vi "SetActiveScanFunc.vi"(4 "FuncIndex":i32, 6 "SingleParMode":bool, 8 "error in (no error)":errorcluster caption="entrée d'erreur (pas d'erreur)", 9 "ScanTag":string, 10 "ScanTreeRef":refnum<vi>, 11 "Experiment en entrée":refnum<class "Experiment.lvclass"> caption="DNL_LabVIEW Object in") -> (0 "error out":errorcluster caption="sortie d'erreur", 1 "DesactivatedSPM":bool, 2 "SingleParModeOut":bool, 3 "Experiment en sortie":refnum<class "Experiment.lvclass"> caption="DNL_LabVIEW Object out")   [LabVIEW 2019, in "Experiment.lvclass"]
uses:
  Experiment.lvclass
  Experiment.lvclass/Experiment.ctl
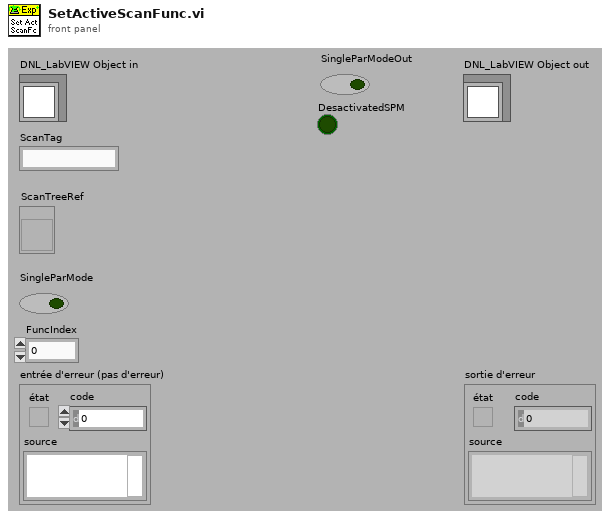
[diagram p1: front panel]
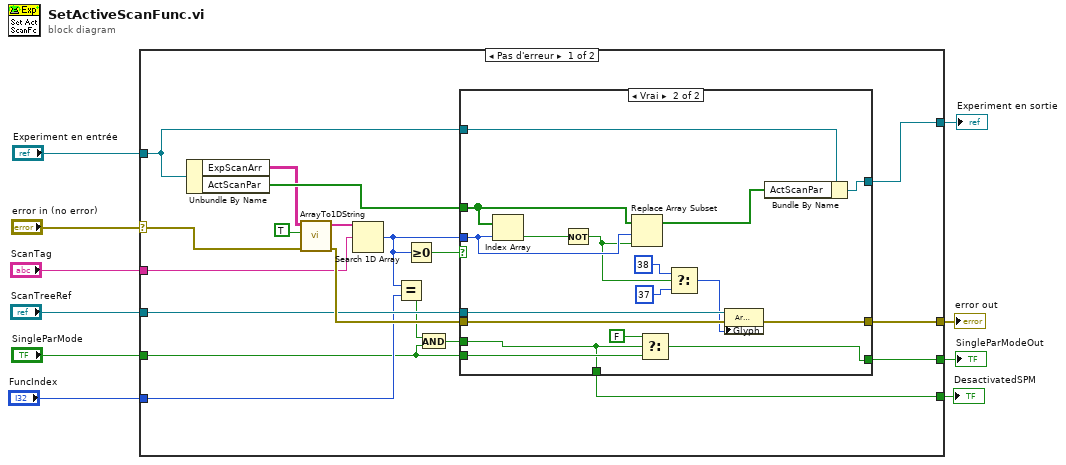
[diagram p0: block diagram]
diagram:
  n1 = case shown="Pas d'erreur" "error in (no error)" {
    selector: "error in (no error)" -> [w22 w52]
    tunnel: [w21 w52] -> w9
    tunnel: [w18 w51] -> w7
    tunnel: "Experiment en entrée" -> [w24 w51]
    tunnel: "ScanTag" -> [w25 _]
    tunnel: "ScanTreeRef" -> [w23 _]
    tunnel: "FuncIndex" -> [w16 _]
    tunnel: "SingleParMode" -> [w12 w50]
    tunnel: [w13 w50] -> w2
    tunnel: [w11 _] -> w1
    frame No Error {
      n2 = Unbundle By Name(w24) -> ("ExpScanArr"=w19:string[][], "ActScanPar"=w20:bool[])
      n3 = call <userlib>:"ArrayTo1DString.vi"("ErrorIn(No Error)"=w22, "DelArrEnd(F)"=TRUE ("DelArrEnd"), "tableau"=w19) -> ("sortie d'erreur"=w27:errorcluster, "Array Out"=w28:string[])  [unwired: 6 in, 1 out]
      n4 = Search 1D Array(1D array=w28, element=w25) -> (index of element=w17:i32)  [unwired: 1 in]
      n5 = Equal?(x=w17, y=w16) -> (x = y?=w15:bool)
      n6 = Greater Or Equal To 0?(x=w17) -> (x >= 0?=w26:bool)
      n7 = And(x=w15, y=w12) -> (x .and. y?=w14:bool)
      n8 = case shown="Vrai" w26 {
        tunnel: w24 -> [w31 w49]
        tunnel: [w31 w48] -> w18
        tunnel: w23 -> [_ w47]
        tunnel: w20 -> [_ w43]
        tunnel: w17 -> [_ w42]
        tunnel: w27 -> [w32 w40]
        tunnel: [w32 w38] -> w21
        tunnel: w14 -> [_ w33]
        tunnel: [w30 w35] -> w13
        tunnel: w12 -> [w30 w36]
        tunnel: [_ w33] -> w11
        frame False {
        }
        frame True {
          n9 = Index Array(array=w43, index=w42) -> (element=w44:bool)
          n10 = Not(x=w44) -> (.not. x?=w41:bool)
          n11 = Replace Array Subset(array=w43, new element=w41, index=w42) -> (w37:bool[])
          n12 = Select(t=FALSE ("cas vrai"), s=w33, f=w36) -> (s? t:f=w35:bool)
          n13 = Select(t=38, s=w41, f=37) -> (s? t:f=w39:i32)
          n14 = property class="Arbre (strict)"(reference=w47, error in=w40, "Glyph"=w39) -> (error out=w38:errorcluster)  [unwired: 1 out]
          n15 = Bundle By Name(cluster=w49, "ActScanPar"=w37) -> (w48:refnum<class "Experiment.lvclass">)
        }
      }
    }
    frame Error {
    }
  }
  "error out" <- w9
  "Experiment en sortie" <- w7
  "SingleParModeOut" <- w2
  "DesactivatedSPM" <- w1
